vi "Node Operation.vi"(8 "error in (no error)":errorcluster, 9 "Formula Variable Table In":refnum<class "Formula Variable Table.lvclass">, 11 "Formula Phrasing Binary Tree Node in":refnum<class "Formula Phrasing Binary Tree Node.lvclass">) -> (0 "error out":errorcluster, 2 "Value Out":dbl format="%#_f", 3 "Formula Phrasing Binary Tree Node out":refnum<class "Formula Phrasing Binary Tree Node.lvclass">)   [LabVIEW 2024, in "Formula Phrasing Binary Tree Node.lvclass"]
uses:
  Formula Phrasing Binary Tree Node.lvclass
  Formula Phrasing Binary Tree Node.lvclass/Formula Phrasing Binary Tree Node.ctl
  Formula Variable Table/Formula Variable Table.lvclass
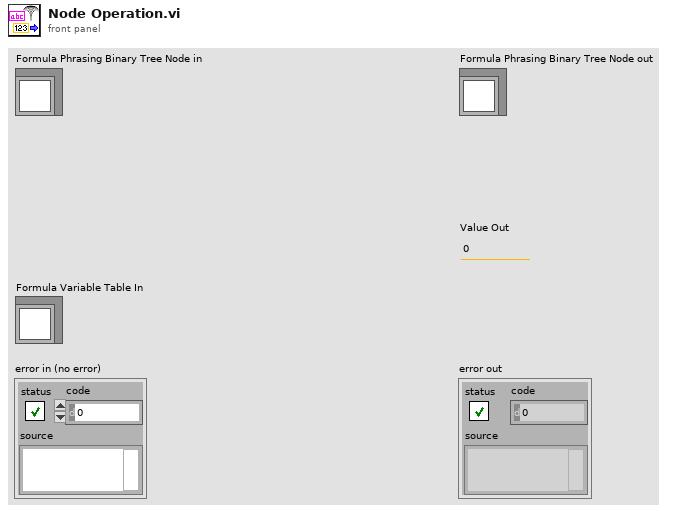
[diagram p1: front panel]
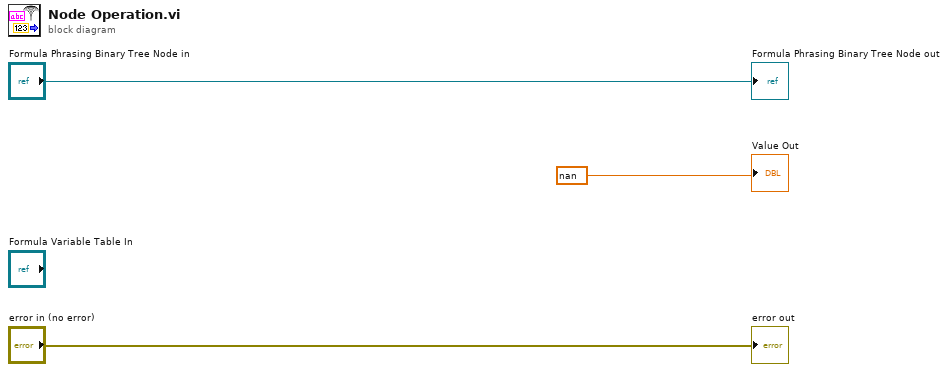
[diagram p0: block diagram]
diagram:
  "error out" <- "error in (no error)"
  "Formula Phrasing Binary Tree Node out" <- "Formula Phrasing Binary Tree Node in"
  "Value Out" <- nan
